vi "BindControlToMatlabValue.vi"(6 "Direction":T1, 8 "AllowVariantValues (f)":bool, 9 "Controls[]":refnum<vi>[](array[refnum]), 10 "Control":refnum<vi>, 11 "ExpID":string) -> (3 "Bound Events":T2[](array[typedef]))   [LabVIEW 2017]
uses:
  Types/ControlValueChangeEventBindingType.ctl
  Types/MatlabBindingDirectionEnum.ctl
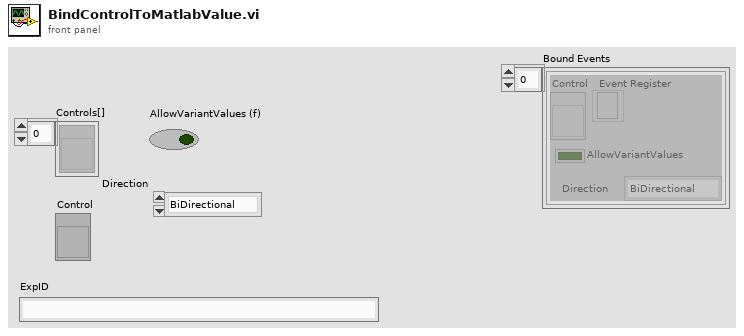
[diagram p1: front panel]
types:
  T1 = typedef "MatlabBindingDirectionEnum.ctl" = enum16{"BiDirectional", "FromMatlab", "ToMatlab"}
  T2 = typedef "ControlValueChangeEventBindingType.ctl" = cluster{"Control":refnum<vi>, "Event Register":refnum<event-registration>, "AllowVariantValues":bool, "Direction":T1}
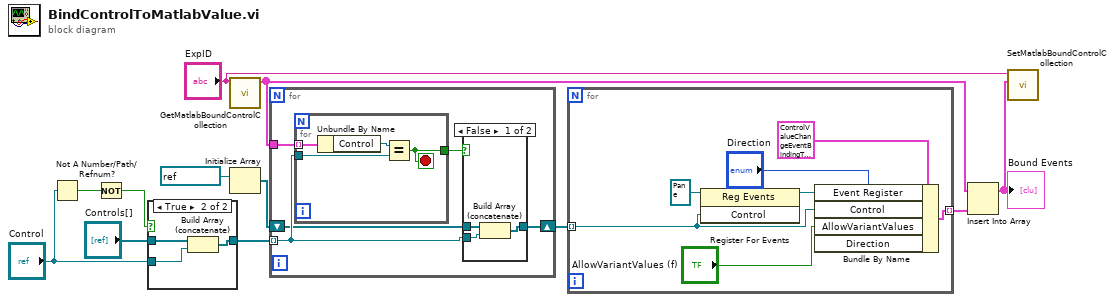
[diagram p0: block diagram]
diagram:
  n1 = Not A Number/Path/Refnum?(number/path/refnum="Control") -> (NaN/Path/Refnum?=w12:bool)
  n2 = Not(x=w12) -> (.not. x?=w1:bool)
  n3 = case shown="True" w1 {
    tunnel: "Controls[]" -> [w13 w16]
    tunnel: "Control" -> [_ w15]
    tunnel: [w13 w14] -> w9
    frame False {
    }
    frame True {
      n4 = Build Array (concatenate)(w16, w15) -> (w14:refnum<vi>[])
    }
  }
  n5 = call "GetMatlabBoundControlCollection.vi"("ExpID"="ExpID") -> ("Bound Controls"=w8:T2[])  [unwired: 10 in]
  n6 = Initialize Array(refnum<vi> refnum ("Control")) -> (w2:refnum<vi>[])  [unwired: 1 in]
  n7 = for {
    tunnel: w9 -> [w20] mode=indexing
    tunnel: w8 -> [w21]
    shift-right: [w17] -> w4
    shift-left: w2 -> [w19]
    n8 = for {
      tunnel: w21 -> [w29] mode=indexing
      tunnel: w20 -> [w27]
      tunnel: [w26] -> w18
      stop <- w26 stop-if-true
      n9 = Unbundle By Name(w29) -> ("Control"=w28:refnum<vi>)
      n10 = Equal?(x=w28, y=w27) -> (x = y?=w26:bool)
    }
    n11 = case shown="False" w18 {
      tunnel: w20 -> [w24 _]
      tunnel: w19 -> [w23 w25]
      tunnel: [w22 w25] -> w17
      frame False {
        n12 = Build Array (concatenate)(w23, w24) -> (w22:refnum<vi>[])
      }
      frame True {
      }
    }
  }
  n13 = for {
    tunnel: [w33] -> w7 mode=indexing
    tunnel: w4 -> [w32] mode=indexing
    n14 = register-events(reference=refnum<event-registration> refnum ("event registration refnum"), w32) -> (reference out=w34:refnum<event-registration>)  [unwired: 1 in, 1 out]
    n15 = Bundle By Name(cluster=T2 {"Control"=refnum, "Event Register"=refnum, "AllowVariantValues"=FALSE, "Direction"=enum."BiDirectional"}, "Event Register"=w34, "Control"=w32, "AllowVariantValues"="AllowVariantValues (f)", "Direction"="Direction") -> (w33:T2)
  }
  n16 = Insert Into Array(array=w8, new element=w7) -> (w6:T2[])  [unwired: 1 in]
  "Bound Events" <- w6
  n17 = call "SetMatlabBoundControlCollection.vi"("Bound controls"=w6, "ExpID"="ExpID") -> ()  [unwired: 10 in]
